vi "VisualInspection.vi"(8 "error in (no error)":errorcluster, 11 "TableRef":refnum<vi>) -> (0 "error out":errorcluster)   [LabVIEW 2017]
panel:
  in  "Cancel Button":bool
  in  "OK Button":bool
  in  "7.5.1.1":bool
  in  "7.3":bool
  in  "7.2.3":bool
  in  "7.2.4":bool
  in  "7.2.5":bool
  in  "6.2.2.1":bool
  in  "6.2.2.2":bool
  in  "6.2.2.3":bool
  in  "6.2.2.4":bool
  in  "7.1":bool
  in  "6.2.1.1":bool
  in  "7.2.2":bool
  in  "6.1.2":bool
  in  "7.2.1.1":bool
  in  "7.2.1":bool
  in  "6.1.1":bool
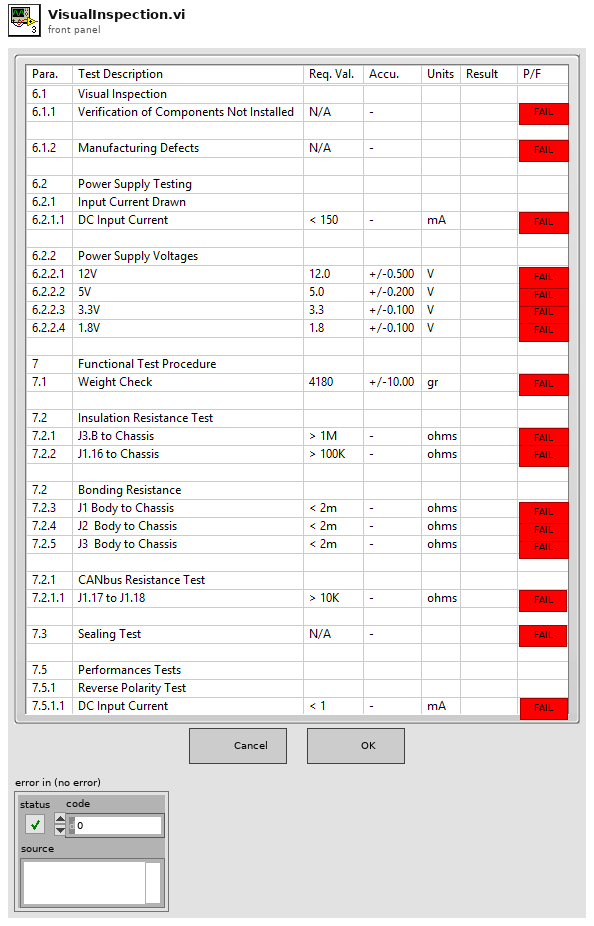
[diagram p1: front panel]
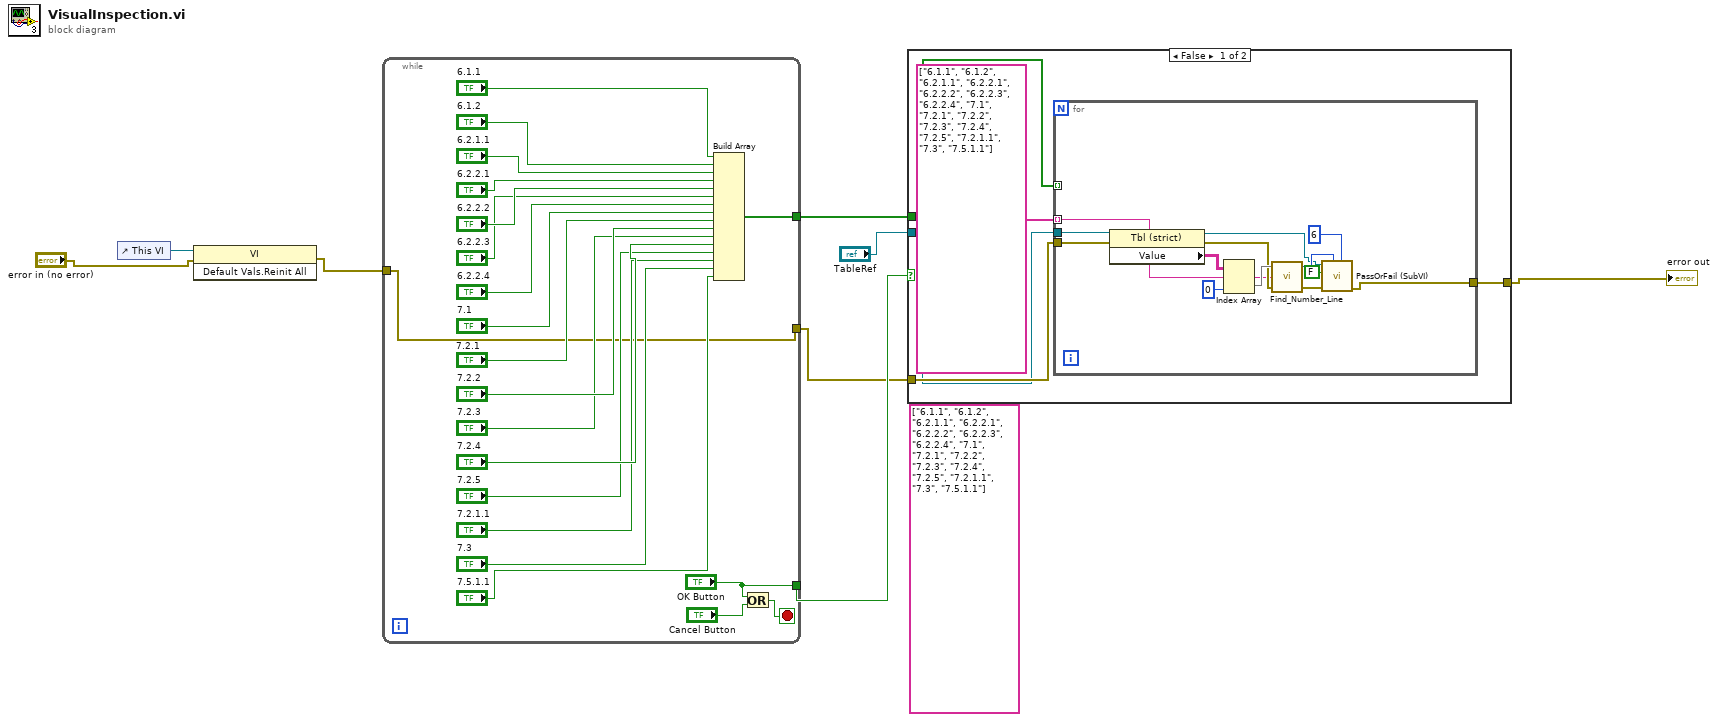
[diagram p0: block diagram]
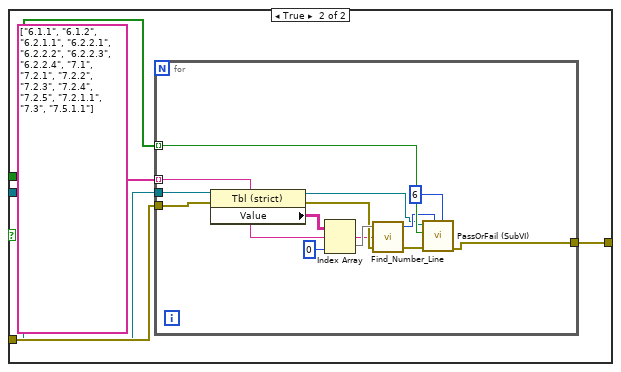
[diagram p2: hidden frame]
diagram:
  (unwired) string[] ["6.1.1", "6.1.2", "6.2.1.1", "6.2.2.1", "6.2.2.2", "6.2.2.3", "6.2.2.4", "7.1", "7.2.1", "7.2.2", "7.2.3", "7.2.4", "7.2.5", "7.2.1.1", "7.3", "7.5.1.1"]
  n1 = control-ref of="This VI"() -> (w3:refnum<vi>)
  n2 = invoke class="VI" method="Default Vals.Reinit All"(reference=w3, error in="error in (no error)") -> (error out=w8:errorcluster)  [unwired: 1 in, 2 out]
  n3 = while {
    tunnel: w8 -> [w9]
    tunnel: [w11] -> w7
    tunnel: ["OK Button"] -> w6
    tunnel: [w9] -> w5
    stop <- w28 stop-if-true
    n4 = Build Array("6.1.1", "6.1.2", "6.2.1.1", "6.2.2.1", "6.2.2.2", "6.2.2.3", "6.2.2.4", "7.1", "7.2.1", "7.2.2", "7.2.3", "7.2.4", "7.2.5", "7.2.1.1", "7.3", "7.5.1.1") -> (w11:bool[])
    n5 = Or(x="OK Button", y="Cancel Button") -> (x .or. y?=w28:bool)
  }
  n6 = case shown="False" w6 {
    tunnel: w7 -> [w33 w51]
    tunnel: w5 -> [w32 w50]
    tunnel: [w31 w49] -> w1
    tunnel: "TableRef" -> [w30 w48]
    frame False {
      n7 = for {
        tunnel: string[] ["6.1.1", "6.1.2", "6.2.1.1", "6.2.2.1", "6.2.2.2", "6.2.2.3", "6.2.2.4", "7.1", "7.2.1", "7.2.2", "7.2.3", "7.2.4", "7.2.5", "7.2.1.1", "7.3", "7.5.1.1"] -> [w43] mode=indexing
        tunnel: w33 -> [_] mode=indexing
        tunnel: w32 -> [w38]
        tunnel: [w37] -> w31
        tunnel: w30 -> [w36]
        n8 = property class="Tbl (strict)"(reference=w36, error in=w38) -> (reference out=w39:refnum<vi>, error out=w44:errorcluster, "Value"=w47:string[][])
        n9 = Index Array(array=w47, index (col)=0 ("disabled index (col)")) -> (element=w45:string[])  [unwired: 1 in]
        n10 = call "Find_Number_Line.vi"("error in"=w44, "Test Paragraph"=w43, "Row Headers[]"=w45) -> ("error out"=w42:errorcluster, "Line number"=w41:i32)  [unwired: 1 out]
        n11 = call "PassOrFail (SubVI).vi"("disabled index (col)"=6, "index (row)"=w41, "error in (no error)"=w42, "Boolean"=FALSE, "Table in"=w39) -> ("error out"=w37:errorcluster)  [unwired: 6 in]
      }
    }
    frame True {
      n12 = for {
        tunnel: string[] ["6.1.1", "6.1.2", "6.2.1.1", "6.2.2.1", "6.2.2.2", "6.2.2.3", "6.2.2.4", "7.1", "7.2.1", "7.2.2", "7.2.3", "7.2.4", "7.2.5", "7.2.1.1", "7.3", "7.5.1.1"] -> [w61] mode=indexing
        tunnel: w51 -> [w59] mode=indexing
        tunnel: w50 -> [w55]
        tunnel: [w54] -> w49
        tunnel: w48 -> [w53]
        n13 = property class="Tbl (strict)"(reference=w53, error in=w55) -> (reference out=w56:refnum<vi>, error out=w62:errorcluster, "Value"=w65:string[][])
        n14 = Index Array(array=w65, index (col)=0 ("disabled index (col)")) -> (element=w63:string[])  [unwired: 1 in]
        n15 = call "Find_Number_Line.vi"("error in"=w62, "Test Paragraph"=w61, "Row Headers[]"=w63) -> ("error out"=w60:errorcluster, "Line number"=w58:i32)  [unwired: 1 out]
        n16 = call "PassOrFail (SubVI).vi"("disabled index (col)"=6, "index (row)"=w58, "error in (no error)"=w60, "Boolean"=w59, "Table in"=w56) -> ("error out"=w54:errorcluster)  [unwired: 6 in]
      }
    }
  }
  "error out" <- w1
